vi "_시리얼_Mark10-데이터 수신 (게이지).vi"(5 "시리얼 포트":refnum<visa-resource-name>="COM5") -> (0 "데이터(lb)":dbl format="%.4f", 1 "수신 정상":bool, 2 "시리얼 포트 out":refnum<visa-resource-name>="COM5")   [LabVIEW 2015]
panel:
  out "Process Time(ms)":u32
  out "버퍼 읽기":string
  # "MARK10 게이지 데이터 수신"
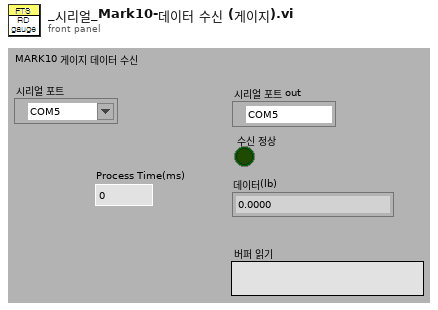
[diagram p1: front panel]
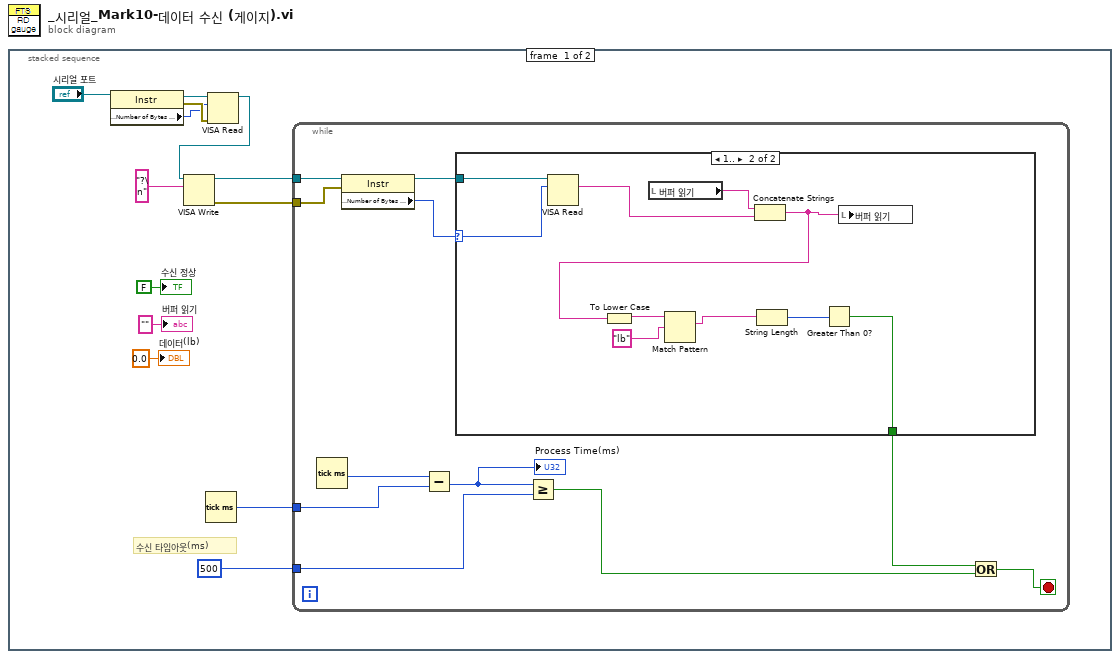
[diagram p0: block diagram]
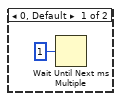
[diagram p2: hidden frame]
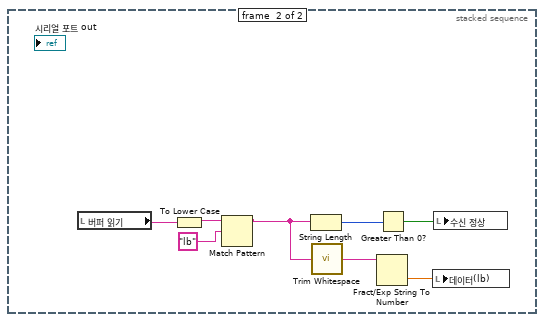
[diagram p3: hidden frame]
diagram:
  n1 = stacked-sequence {
    frame #0 {
      # "수신 타임아웃(ms)"
      n2 = property class="Instr"(reference="시리얼 포트") -> (reference out=w7:refnum<visa-resource-name>, error out=w5:errorcluster, "Serial Settings:Number of Bytes at Serial Port"=w1:u32)  [unwired: 1 in]
      n3 = Tick Count (ms)() -> (millisecond timer value=w9:u32)
      n4 = VISA Read(VISA resource name=w7, byte count=w1, error in (no error)=w5) -> (VISA resource name out=w4:refnum<visa-resource-name>)  [unwired: 3 out]
      n5 = VISA Write(VISA resource name=w4, write buffer="?\n") -> (VISA resource name out=w11:refnum<visa-resource-name>, error out=w10:errorcluster)  [unwired: 1 in, 1 out]
      n6 = while {
        tunnel: w11 -> [w23]
        tunnel: w10 -> [w22]
        tunnel: w9 -> [w19]
        tunnel: 500 -> [w17]
        stop <- w15 stop-if-true
        n7 = Tick Count (ms)() -> (millisecond timer value=w20:u32)
        n8 = property class="Instr"(reference=w23, error in=w22) -> (reference out=w24:refnum<visa-resource-name>, "Serial Settings:Number of Bytes at Serial Port"=w21:u32)  [unwired: 1 out]
        n9 = Subtract(x=w20, y=w19) -> (x-y=w18:u32)
        "Process Time(ms)" <- w18
        n10 = case shown="1.." w21 {
          selector: w21 -> [_ w27]
          tunnel: w24 -> [_ w35]
          tunnel: [_ w28] -> w14
          frame 0, Default {
            n11 = Wait Until Next ms Multiple(millisecond multiple=u32 1 ("ms 배수")) -> ()  [unwired: 1 out]
          }
          frame 1.. {
            n12 = VISA Read(VISA resource name=w35, byte count=w27) -> (read buffer=w33:string)  [unwired: 1 in, 3 out]
            n13 = local read "버퍼 읽기"() -> (w34:string)
            n14 = Concatenate Strings(w34, w33) -> (w32:string)
            n15 = To Lower Case(string=w32) -> (all lower case string=w31:string)
            n16 = Match Pattern(string=w31, regular expression="lb" ("문자열")) -> (match substring=w26:string)  [unwired: 1 in, 3 out]
            n17 = String Length(string=w26) -> (length=w29:i32)
            n18 = Greater Than 0?(x=w29) -> (x > 0?=w28:bool)
            n19 = local write "버퍼 읽기"(w32) -> ()
          }
        }
        n20 = Greater Or Equal?(x=w18, y=w17) -> (x >= y?=w16:bool)
        n21 = Or(x=w14, y=w16) -> (x .or. y?=w15:bool)
      }
      "수신 정상" <- FALSE ("수신 정상")
      "버퍼 읽기" <- "" ("버퍼 읽기")
      "데이터(lb)" <- 0.0 ("데이터(lb)")
    }
    frame #1 {
      n22 = local read "버퍼 읽기"() -> (w37:string)
      n23 = To Lower Case(string=w37) -> (all lower case string=w39:string)
      n24 = Match Pattern(string=w39, regular expression="lb" ("문자열")) -> (before substring=w36:string)  [unwired: 1 in, 3 out]
      n25 = String Length(string=w36) -> (length=w40:i32)
      n26 = call <vilib>:"Trim Whitespace.vi"("string"=w36) -> ("trimmed string"=w43:string)  [unwired: 1 in]
      n27 = Fract/Exp String To Number(string=w43) -> (number=w42:dbl)  [unwired: 3 in, 1 out]
      n28 = Greater Than 0?(x=w40) -> (x > 0?=w41:bool)
      n29 = local write "데이터(lb)"(w42) -> ()
      n30 = local write "수신 정상"(w41) -> ()
    }
  }
